vi "gratebar defects finding sim.vi"(0 "src img path":path, 1 "img out path":path, 2 "threshoulds array":dbl[](array[numeric]), 3 "size":dbl, 5 "error in (no error)":errorcluster) -> (14 "defect ratio":dbl, 15 "frame statue":dbl, 16 "defect type":dbl, 17 "Image Out (duplicate)":T1, 18 "defect ratio 2":dbl, 19 "error out":errorcluster)   [LabVIEW 2019]
uses:
  <vilib>/vision/Image Controls.llb/IMAQ Image.ctl
panel:
  out "Image":T1(plugin-control)
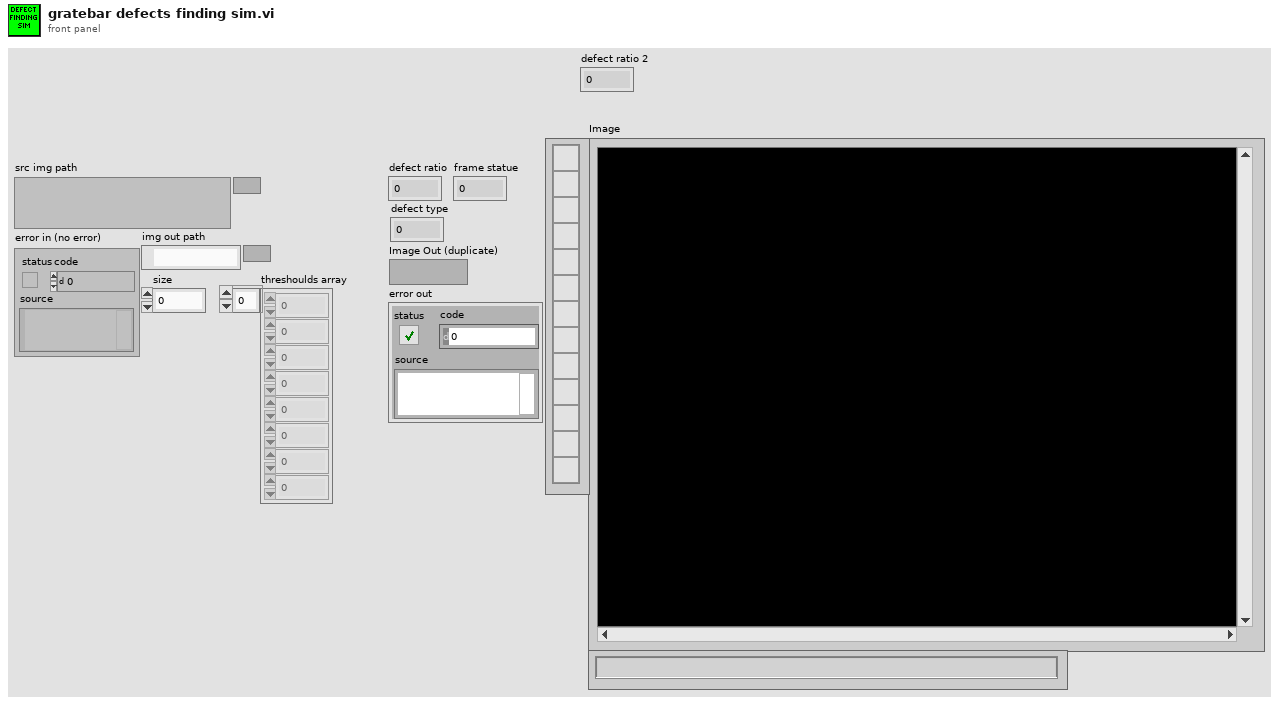
[diagram p1: front panel]
types:
  T1 = typedef "IMAQ Image.ctl" = refnum<image>
  T2 = typedef "Image Type" = u32
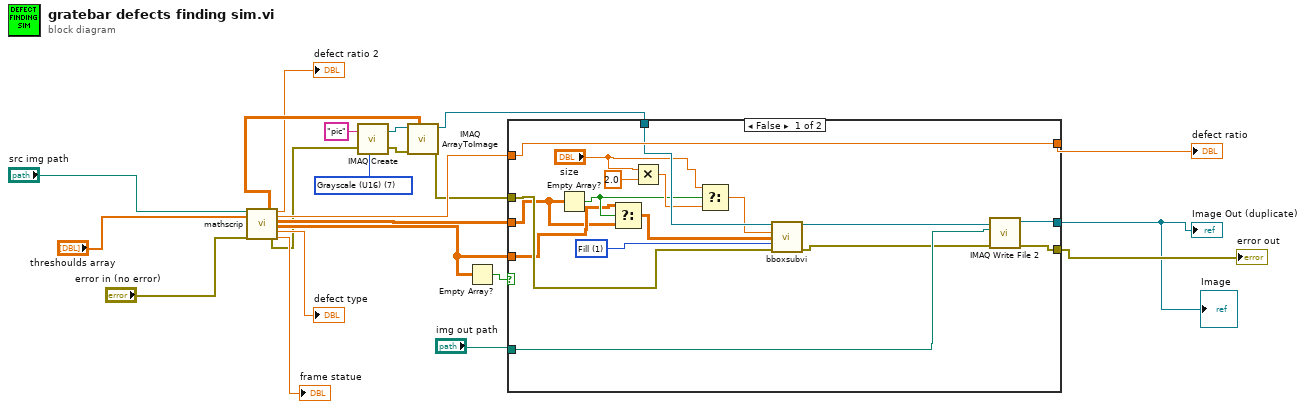
[diagram p0: block diagram]
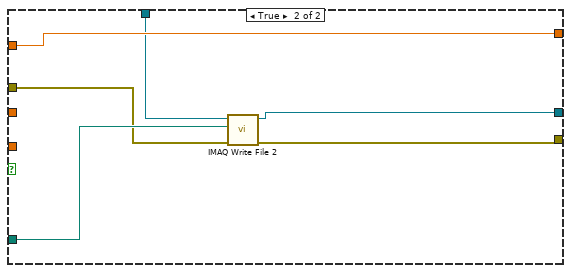
[diagram p2: hidden frame]
diagram:
  w11 = T2 7 items=["Grayscale (U8)", "Grayscale (I16)", "Grayscale (SGL)", "Complex (CSG)", "RGB (U32)", "HSL (U32)", "RGB (U64)", "Grayscale (U16)"] ("Image Type")
  n1 = call "mathscrip.vi"("image path"="src img path", "threshoulds array"="threshoulds array", "error in"="error in (no error)") -> ("imgout"=w7:dbl[][], "error out"=w6:errorcluster, "defect ratio 2"=→"defect ratio 2":dbl, "defect ratio1"=w18:dbl, "damage points 2"=w15:dbl[][], "damage points"=w17:dbl[][], "defect type"=→"defect type":dbl, "frame statue"=→"frame statue":dbl)  [unwired: 9 in]
  n2 = call "IMAQ Create"("Image Name"="pic", "Image Type"=w11, "error in (no error)"=w6) -> ("New Image"=w8:T1, "error out"=w9:errorcluster)  [unwired: 2 in]
  n3 = call "IMAQ ArrayToImage"("Image Pixels (U16)"=w7, "error in (no error)"=w9, "Image"=w8) -> ("error out"=w5:errorcluster, "Image Out"=w4:T1)  [unwired: 7 in]
  n4 = Empty Array?(array=w17) -> (empty?=w22:bool)
  n5 = case shown="False" w22 {
    tunnel: [w33 w42] -> w19
    tunnel: w17 -> [w27 _]
    tunnel: "img out path" -> [w35 w44]
    tunnel: [w34 w43] -> w2
    tunnel: w18 -> [w39 w45]
    tunnel: [w39 w45] -> w20
    tunnel: w15 -> [w26 _]
    tunnel: w5 -> [w36 w41]
    tunnel: w4 -> [w37 w40]
    frame False {
      w38 = u32 1 items=["Frame", "Fill"] ("Drawing Mode (Frame)")
      n6 = Empty Array?(array=w26) -> (empty?=w28:bool)
      n7 = Select(t=w27, s=w28, f=w26) -> (s? t:f=w25:dbl[][])
      n8 = Multiply(x="size", y=2.0) -> (x*y=w31:dbl)
      n9 = Select(t="size", s=w28, f=w31) -> (s? t:f=w30:dbl)
      n10 = call "bboxsubvi.vi"("Image"=w37, "size"=w30, "array"=w25, "Drawing Mode (Frame)"=w38, "error in"=w36) -> ("Image Out"=w24:T1, "error out"=w23:errorcluster)  [unwired: 9 in]
      n11 = call-poly "IMAQ Write File 2"("error in (no error)"=w23, "File Path"=w35, "Image"=w24) -> ("error out"=w33:errorcluster, "Image Out (duplicate)"=w34:T1)  [unwired: 7 in]
    }
    frame True {
      n12 = call-poly "IMAQ Write File 2"("error in (no error)"=w41, "File Path"=w44, "Image"=w40) -> ("error out"=w42:errorcluster, "Image Out (duplicate)"=w43:T1)  [unwired: 7 in]
    }
  }
  "defect ratio" <- w20
  "Image Out (duplicate)" <- w2
  "error out" <- w19
  "Image" <- w2
